vi "Parse.vi"(8 "Error In":errorcluster, 11 "object in":refnum<class "2025_1.lvclass">) -> (0 "Error Out":errorcluster, 3 "object out":refnum<class "2025_1.lvclass">)   [LabVIEW 2025, in "2025_1.lvclass"]
uses:
  2025_1.lvclass
  Turns.ctl
  Direction.ctl
  2025_1.lvclass/2025_1.ctl
  <vilib>/Utility/error.llb/Trim Whitespace One-Sided.vi
  <userlib>/_OpenG.lib/string/string.llb/openg_string.lvlib
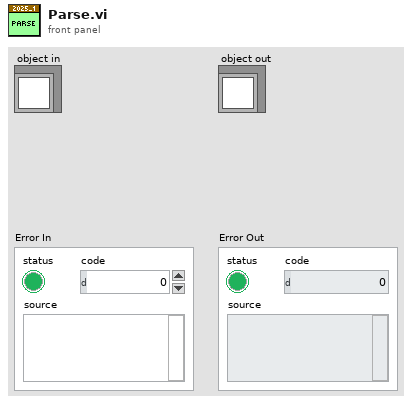
[diagram p1: front panel]
types:
  T1 = typedef "2025_1.lvclass/Turns.ctl" = cluster{"Direction":T2, "Steps":i64}
  T2 = typedef "2025_1.lvclass/Direction.ctl" = enum16{"Left", "Right"}
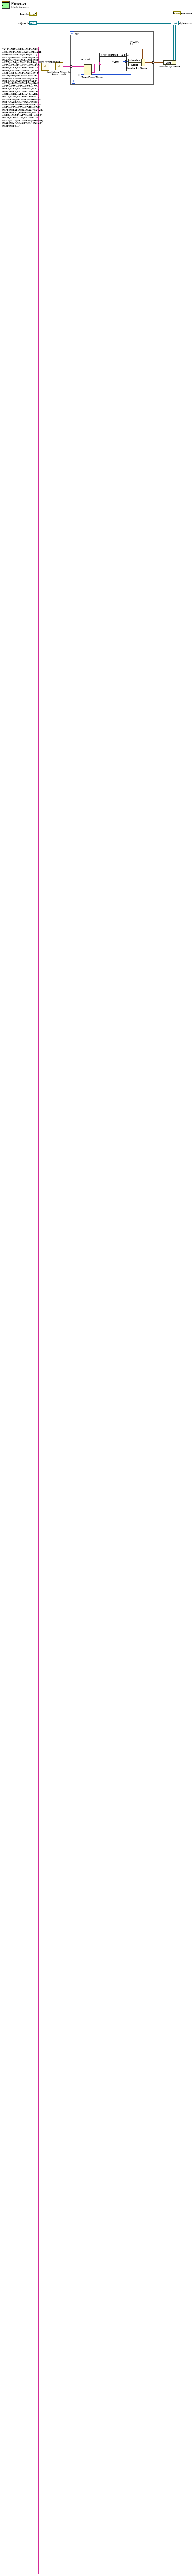
[diagram p0: block diagram]
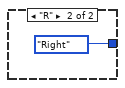
[diagram p2: hidden frame]
diagram:
  n1 = call <vilib>:"Trim Whitespace.vi"("string"="L40\nR27\nR20\nR12\nR28\nL9\nR31\nR45\nL19\nR2\nL25\nL46\nR1\nR26\nL44\nL27\nR11\nR41\nL11\nR14\nR33\nL2\nR24\nL8\nL31\nR3\nR3\nR17\nL14\nL8\nL16\nR44\nL39\nL7\nR2\nL17\nL2\nR33\nR50\nL33\nR45\nL33\nL22\nR35\nR50\nL24\nR47\nL50\nL49\nR14\nR13\nR10\nR45\nR96\nR4\nR29\nL29\nL34\nL66\nL59\nL69\nR18\nR56\nR54\nR5\nL20\nR92\nL38\nR99\nR62\nL87\nR20\nR41\nL97\nL77\nL93\nR85\nL92\nR82\nL82\nR71\nR28\nL94\nL96\nR97\nR10\nL16\nL48\nL52\nR92\nL16\nL44\nL32\nR72\nL10\nR38\nL45\nR17\nR7\nR14\nR7\nL69\nL44\nL87\nR87\nL68\nR24\nL67\nR95\nL60\nL65\nL46\nL603\nR272\nL69\nL93\nL73\nR366\nR76\nL75\nR515\nL96\nL214\nL428\nL55\nR327\nR5\nR10\nR16\nR19\nR176\nL878\nL24\nR59\nR75\nL8\nL720\nR30\nL30\nR87\nL37\nR70\nR96\nR4\nL4\nL23\nR27\nR268\nR64\nL825\nL49\nR94..." ("PuzzleInput")) -> ("trimmed string"=w3:string)  [unwired: 1 in]
  n2 = call <userlib>:"Multi-line String to Array__ogtk.vi"("string"=w3) -> ("lines"=w2:string[])
  n3 = for {
    tunnel: w2 -> [w15] mode=indexing
    tunnel: [w8] -> w1 mode=indexing
    n4 = Scan From String(format string="%1s%d", input string=w15, default 2=i64 0 ("default value 1")) -> (output 1=w12:string, output 2=w10:i64)  [unwired: 3 in, 3 out]
    n5 = case shown="\"L\", Default" w12 {
      tunnel: [Direction."Left" Direction."Right"] -> w11
      frame "L", Default {
      }
      frame "R" {
      }
    }
    n6 = Bundle By Name(cluster=T1 {"Direction"=enum."Left", "Steps"=0} ("output cluster"), "Direction"=w11, "Steps"=w10) -> (w8:T1)
  }
  n7 = Bundle By Name(cluster="object in", "Turns"=w1) -> (→"object out":refnum<class "2025_1.lvclass">)
  "Error Out" <- "Error In"
